vi "var_of_mem.vi"() -> ()   [LabVIEW 2017]
uses:
  <vilib>/Platform/TimedLoop/XDataNode/timing_clust.ctl
  <vilib>/Platform/TimedLoop/XDataNode/nitl_modes.ctl
  <vilib>/Platform/TimedLoop/XDataNode/wakeup.ctl
  <vilib>/rvi/IPIntegrationNode/IPINode_Typedef/niFpgaIPINodeSupportedFamilies.ctl
  <vilib>/rvi/Emulation/niFpgaSctlEmulationGetInTimedLoop.vi
  <vilib>/rvi/Emulation/niFpgaEmulationReportErrorSimple.vi
  <vilib>/rvi/Emulation/niFpgaGetClockAttributes.vi
  <vilib>/rvi/Emulation/niFpgaCriticalErrorInLSC.vi
  <vilib>/rvi/Memory/Memory_Emulation/nirvimemoryFastEmulation.vi
  <vilib>/rvi/Memory/Memory_Emulation/nirvimemoryEmulation.vi
  <vilib>/rvi/Emulation/niFpgaEmulationIsFPGAContextNoSignature.vi
  <vilib>/rvi/DataTransferAndStorage/Container/Common/niFpgaContainerGetUniqueNameForEmu.vi
  <vilib>/rvi/Emulation/niFpgaProcessEmulError.vi
  <vilib>/rvi/errors/nirviReportUnexpectedCaseInternalError (U32).vi
  <vilib>/rvi/IPIntegrationNode/IPINode_Utilities/niFpgaIPINodeSimCore.vi
  <vilib>/platform/TimedLoop/XDataNode/XDataNode.xnode
  <vilib>/rvi/DataTransferAndStorage/Container/XNode/niFpgaContainer.xnode
  <vilib>/rvi/XilinxIP/XIPIN_XNode/niFpgaXIPIN.xnode
  var_of_mem/Multiply Accumulator/Multiply_Accumulator_86883BA6B7704AADBBA8A26EFBF54CC2.dll
  <vilib>/rvi/IPIntegrationNode/IPINode_Xnode/niFpgaIPINode.xnode
  <vilib>/rvi/FXPMathLib/FxpSub/XNode/nifxpmath_Sub.xnode
  <vilib>/Platform/TimedLoop/XDataNode/XDNodeRunTimeDep.lvlib
  <vilib>/rvi/FXPMathLib/sim/FxpSim.dll
panel:
  out "s":fxp<+/-,32,10>
  out "Array":fxp<+/-,32,10>[](array[numeric])
  in  "mean":fxp<+/-,32,21>
  in  "N":u8
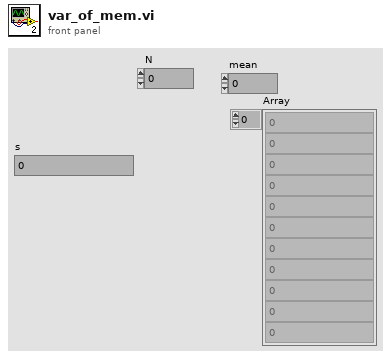
[diagram p1: front panel]
types:
  T1 = typedef "XDNodeRunTimeDep.lvlib/timing_clust.ctl" = cluster{"Expected End [f-1]":u64, "Actual End [f-1]":u64, "Finished Late? [f-1]":bool, "Expected End [i-1]":u64, "Actual End [i-1]":u64, "Finished Late? [i-1]":bool, "Expected Start [i]":u64, "Actual Start [i]":u64, "Expected Start [f]":u64, "Actual Start [f]":u64, "Source Name":string, "Structure Name":string, "Period":i64, "Deadline":i64, "Offset":i64, "Start":i64, "Priority":i32, "Timeout":i32, "Mode":T2, "Wakeup Reason":T3, "Error":errorcluster, "Source Type":string, "Secondary Source Type":string, "Global End Time":u64, "Global Start Time":u64, "Frame Duration":u64, "Iteration Duration":u64, "Assigned CPU":i32, "I/O Scan Engine Mode":u32}
  T2 = typedef "XDNodeRunTimeDep.lvlib/nitl_modes.ctl" = enum32{"No Change", "Process missed periods, maintain original phase", "Discard missed periods, maintain original phase", "Process missed periods, ignore original phase", "Discard missed periods, ignore original phase"}
  T3 = typedef "XDNodeRunTimeDep.lvlib/wakeup.ctl" = enum32{"Normal", "Aborted", "Asynchronous wakeup", "Timing source error", "Timed loop error", "Timeout"}
  T4 = typedef "niFpgaIPINodeSupportedFamilies.ctl" = cluster{"unlimited?":bool, "supported targets":string[]}
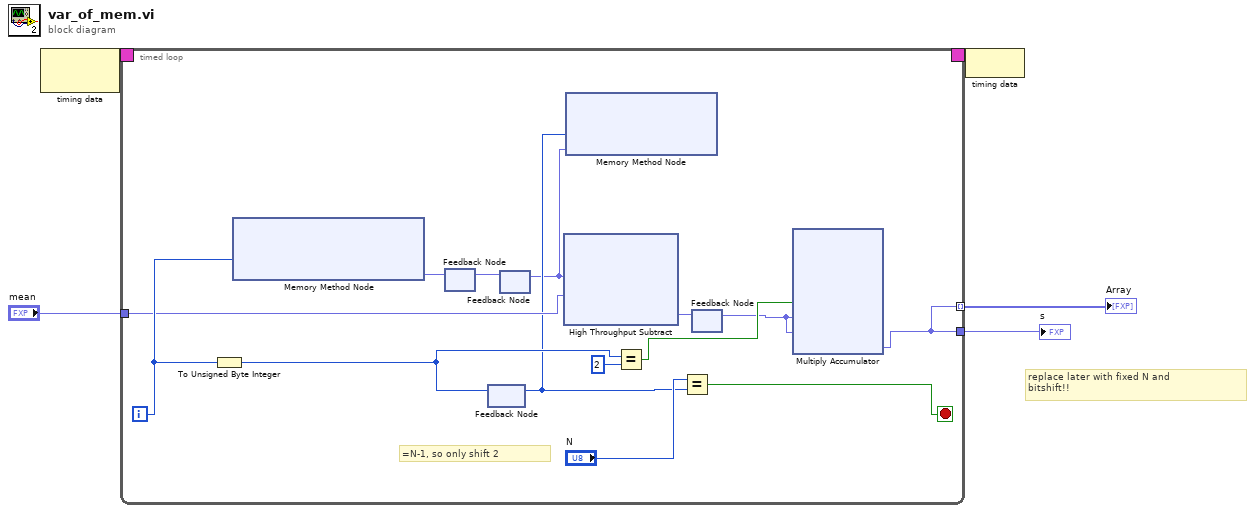
[diagram p0: block diagram]
diagram:
  # "replace later with fixed N and \nbitshift!!"
  n1 = node-c288() -> (w5:T1)  [unwired: 1 in]
  n2 = timed-loop {
    timing: w5 -> [_]
    timing-out: [_] -> w4
    tunnel: [w8] -> w1
    tunnel: "mean" -> [w12]
    tunnel: [w8] -> w2 mode=indexing
    i -> [w15]
    stop <- w16 stop-if-true
    # "=N-1, so only shift 2"
    n3 = To Unsigned Byte Integer(number=w15) -> (unsigned 8bit integer=w14:u8)
    n4 = xnode ("Memory Method Node")("Address"=w15) -> ("Data"=w19:fxp<+/-,16,5>)  [unwired: 1 in, 1 out]
    n5 = feedback-in #1(w19) -> ()
    n6 = feedback #1() -> (w18:fxp<+/-,16,5>)  [unwired: 1 in]
    n7 = feedback #2() -> (w7:u8)  [unwired: 1 in]
    n8 = feedback-in #2(w14) -> ()
    n9 = feedback #3() -> (w6:fxp<+/-,16,5>)  [unwired: 1 in]
    n10 = feedback-in #3(w18) -> ()
    n11 = xnode "High Throughput Subtract"("x"=w6, "y"=w12) -> ("x-y"=w13:fxp<+/-,33,22>)
    n12 = xnode ("Memory Method Node")("Address"=w7, "Data"=w6) -> ()  [unwired: 1 in, 1 out]
    n13 = Equal?(x=w14, y=u8 2) -> (x = y?=w10:bool)
    n14 = Equal?(x="N", y=w7) -> (x = y?=w16:bool)
    n15 = feedback #4() -> (w9:fxp<+/-,33,22>)  [unwired: 1 in]
    n16 = feedback-in #4(w13) -> ()
    n17 = xnode ("Multiply Accumulator")("sclr"=w10, "a"=w9, "b"=w9) -> ("s"=w8:fxp<+/-,48,26>)  [unwired: 2 in]
  }
  "Array" <- w2
  "s" <- w1
  n18 = node-c288(w4) -> ()
